vi "Destroy User Events.vi"(11 "Nested in":refnum<class "RefNums and UICtrl.lvclass">) -> (3 "Nested out":refnum<class "RefNums and UICtrl.lvclass">)   [LabVIEW 2020, in "RefNums and UICtrl.lvclass"]
uses:
  RefNums and UICtrl.lvclass
  RefNums and UICtrl.lvclass/RefNums and UICtrl.ctl
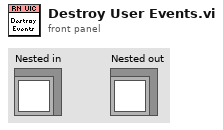
[diagram p1: front panel]
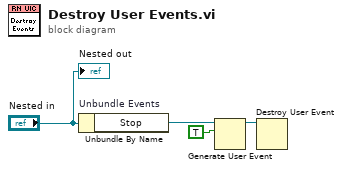
[diagram p0: block diagram]
diagram:
  n1 = Unbundle By Name "Unbundle Events"("Nested in") -> ("Stop"=w2:refnum<user-event>)
  n2 = Generate User Event(user event=w2, event data cluster=TRUE ("event data")) -> (user event out=w3:refnum<user-event>)  [unwired: 2 in, 1 out]
  n3 = Destroy User Event(user event=w3) -> ()  [unwired: 1 in, 1 out]
  "Nested out" <- "Nested in"
